vi "robot.vi"() -> ()   [LabVIEW 2016]
panel:
  out "k2":dbl
  out "k1":dbl
  out "sinQ2":dbl
  out "cosQ2":dbl
  in  "y koordinatı":dbl
  in  "x koordinatı":dbl
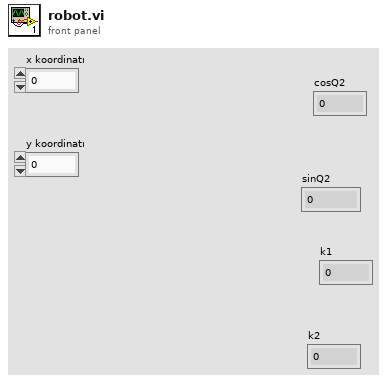
[diagram p1: front panel]
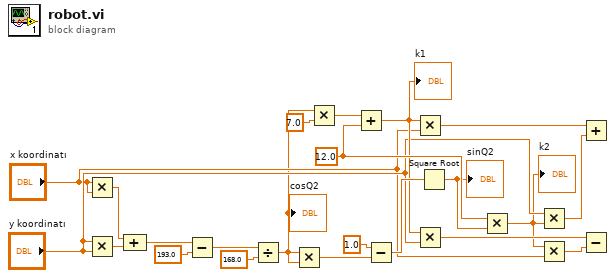
[diagram p0: block diagram]
diagram:
  w11 = 12.0 ("y")
  n1 = Multiply(x="x koordinatı", y="x koordinatı") -> (x*y=w22:dbl)
  n2 = Multiply(x="y koordinatı", y="y koordinatı") -> (x*y=w21:dbl)
  n3 = Compound Arithmetic op=ADD(w22, w21) -> (w20:dbl)
  n4 = Subtract(x=w20, y=193.0) -> (x-y=w18:dbl)
  n5 = Divide(x=w18, y=168.0) -> (x/y=w1:dbl)
  "cosQ2" <- w1
  n6 = Multiply(x=w1, y=w1) -> (x*y=w15:dbl)
  n7 = Multiply(x=w1, y=7.0) -> (x*y=w13:dbl)
  n8 = Add(x=w13, y=w11) -> (x+y=w8:dbl)
  "k1" <- w8
  n9 = Subtract(x=1.0, y=w15) -> (x-y=w14:dbl)
  n10 = Multiply(x=w8, y="x koordinatı") -> (x*y=w10:dbl)
  n11 = Multiply(x=w8, y="y koordinatı") -> (x*y=w6:dbl)
  n12 = Square Root(x=w14) -> (sqrt(x)=w2:dbl)
  "sinQ2" <- w2
  n13 = Multiply(x=w11, y=w2) -> (x*y=w4:dbl)
  "k2" <- w4
  n14 = Multiply(x="y koordinatı", y=w4) -> (x*y=w9:dbl)
  n15 = Multiply(x=w4, y="x koordinatı") -> (x*y=w5:dbl)
  n16 = Add(x=w10, y=w9) -> ()  [unwired: 1 out]
  n17 = Subtract(x=w6, y=w5) -> ()  [unwired: 1 out]
